vi "Motor Control.vi"(0 "GEA2 Reference In":refnum<k24>, 5 "Motor Control":T1={"Speed (RPM)"=0, "Motor Profile Mode"=0, "Acceleration"=10, "Angle (Degrees)"=360, "Amplitude (%)\n-CCW +CW"=100} {"Amplitude (%)\n-CCW +CW" min=-100 max=100 step=5; "Acceleration" min=-400 max=400 step=10; "Motor Profile Mode" items=["Closed Loop", "Not Implemented", "Open Loop ", "Open Loop Angle ", "Coasting", "Braking", "Idle"]; "Speed (RPM)" min=-900 max=0 step=10}, 7 "Action":enum16{"Start", "Stop"}(ring), 11 "Error In":errorcluster) -> (4 "GEA2 Reference Out":refnum<k24>, 15 "Error Out":errorcluster)   [LabVIEW 2018, in "TLMB.lvlib"]
uses:
  Projects/TLMB.lvlib
  D:/Common/LabVIEW GEA2 Toolkit/source/GEA3 DLL Source/GeaCommunication.dll
  Common/LabVIEW GEA2 Toolkit/source/GEA3 DLL Source/GeaCommunication.dll
  type defs/Motor Control Without Stop Start.ctl
  Common/LabVIEW GEA2 Toolkit/GEA3/type defs/Source_Destination.ctl
  Common/LabVIEW GEA2 Toolkit/GEA3/type defs/ERD Write Data In.ctl
  Common/LabVIEW GEA2 Toolkit/GEA3/type defs/Data Type.ctl
  C:/Users/iallatyp/Desktop/New folder/GEA3/library/GEA2_Toolkit.lvlib
panel:
  in  "Standalone?":bool
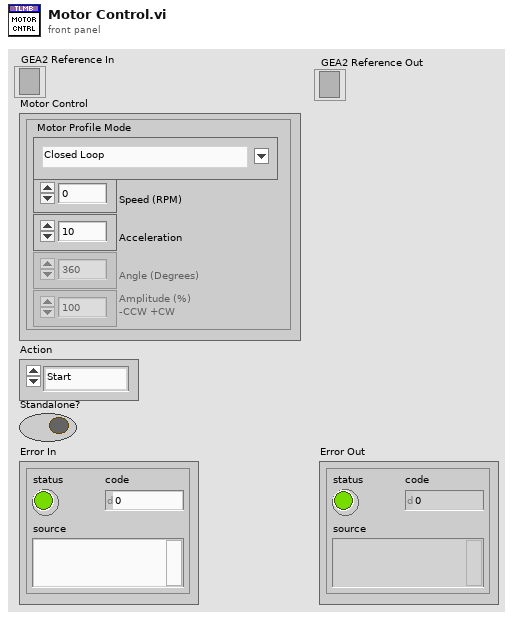
[diagram p1: front panel]
types:
  T1 = typedef "TLMB.lvlib/Motor Control Without Stop Start.ctl" = cluster{"Speed (RPM)":i16, "Motor Profile Mode":u16, "Acceleration":i16, "Angle (Degrees)":i16, "Amplitude (%)\n-CCW +CW":i16}
  T2 = typedef "GEA2_Toolkit.lvlib/ERD Write Data In.ctl" = cluster{"ERD Number":u16, "Data Type":T3, "Data":string}
  T3 = typedef "GEA2_Toolkit.lvlib/Data Type.ctl" = enum16{"string", "boolean", "uint8_t", "uint16_t", "uint32_t", "uint64_t", "int8_t", "int16_t", "int32_t", "int64_t"}
  T4 = typedef "GEA2_Toolkit.lvlib/Source_Destination.ctl" = cluster{"Source":u8, "Destination":u8}
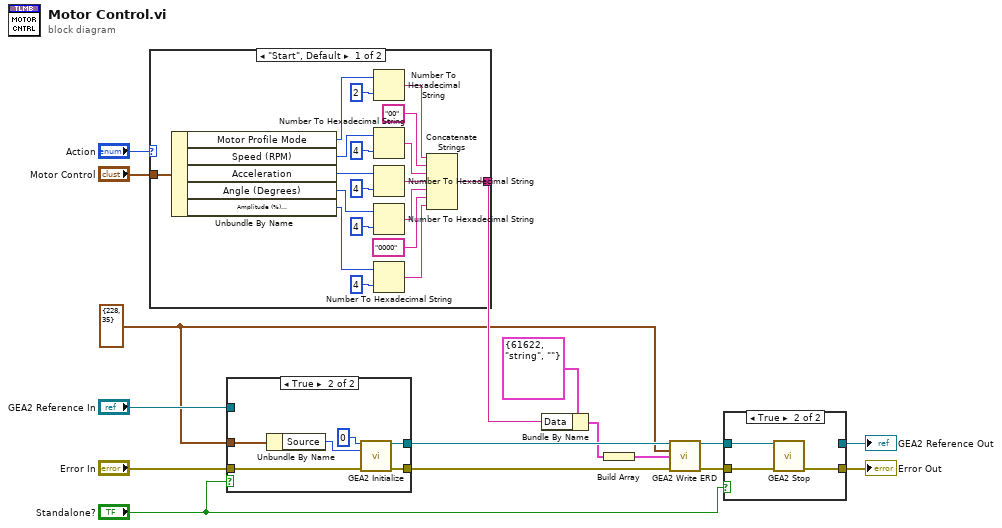
[diagram p0: block diagram]
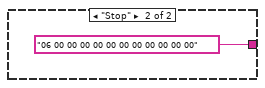
[diagram p2: hidden frame]
diagram:
  w4 = T4 {"Source"=228, "Destination"=35} ("GEA Inputs")
  n1 = case shown="\"Start\", Default" "Action" {
    tunnel: [w35 "06 00 00 00 00 00 00 00 00 00 00 00" ("string")] -> w16
    tunnel: "Motor Control" -> [w18 _]
    frame "Start", Default {
      n2 = Unbundle By Name(w18) -> ("Motor Profile Mode"=w22:u16, "Speed (RPM)"=w17:i16, "Acceleration"=w21:i16, "Angle (Degrees)"=w20:i16, "Amplitude (%)\n-CCW +CW"=w19:i16)
      n3 = Number To Hexadecimal String(1:i16 2 ("width (-)"), 2:w22) -> (0:w33:string)
      n4 = Number To Hexadecimal String(1:i16 4 ("width (-)"), 2:w17) -> (0:w32:string)
      n5 = Number To Hexadecimal String(1:i16 4 ("width (-)"), 2:w21) -> (0:w27:string)
      n6 = Number To Hexadecimal String(1:i16 4 ("width (-)"), 2:w20) -> (0:w26:string)
      n7 = Number To Hexadecimal String(1:i16 4 ("width (-)"), 2:w19) -> (0:w25:string)
      n8 = Concatenate Strings(w33, "00" ("string"), w32, w27, w26, "0000" ("string"), w25) -> (w35:string)
    }
    frame "Stop" {
    }
  }
  n9 = case shown="True" "Standalone?" {
    tunnel: "Error In" -> [w37 w44]
    tunnel: [w37 w43] -> w5
    tunnel: "GEA2 Reference In" -> [w38 _]
    tunnel: [w38 w42] -> w6
    tunnel: w4 -> [_ w40]
    frame False {
    }
    frame True {
      n10 = Unbundle By Name(w40) -> ("Source"=w41:u8)
      n11 = call "GEA2 Initialize.vi"("Board Index"=0, "Source Address"=w41, "error in"=w44) -> ("GEA2 Reference Out"=w42:refnum<k24>, "error out"=w43:errorcluster)  [unwired: 10 in, 1 out]
    }
  }
  n12 = Bundle By Name(cluster=T2 {"ERD Number"=61622, "Data Type"=enum."string", "Data"=""} ("ERD Read Data In"), "Data"=w16) -> (w1:T2)
  n13 = Build Array(w1) -> (w14:T2[])
  n14 = call "GEA2 Write ERD.vi"("GEA2 Reference In"=w6, "GEA Inputs"=w4, "Write ERD List"=w14, "Error In"=w5) -> ("GEA2 Reference Out"=w7:refnum<k24>, "Error Out"=w8:errorcluster)  [unwired: 9 in, 1 out]
  n15 = case shown="True" "Standalone?" {
    tunnel: w8 -> [w46 w49]
    tunnel: [w46 w48] -> w13
    tunnel: [w45 _] -> w12
    tunnel: w7 -> [w45 w47]
    frame False {
    }
    frame True {
      n16 = call "GEA2 Stop.vi"("GEA2 Reference In"=w47, "Error In"=w49) -> ("Error Out"=w48:errorcluster)  [unwired: 13 in]
    }
  }
  "Error Out" <- w13
  "GEA2 Reference Out" <- w12
